vi "Key Join.vi"(11 "Key Elements":string[](array[string])) -> (3 "Key":string)   [LabVIEW 2017]
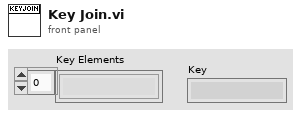
[diagram p1: front panel]
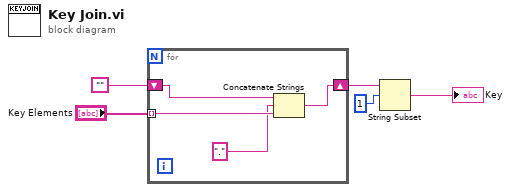
[diagram p0: block diagram]
diagram:
  n1 = for {
    tunnel: "Key Elements" -> [w8] mode=indexing
    shift-right: [w6] -> w3
    shift-left: "" -> [w9]
    n2 = Concatenate Strings(w9, ".", w8) -> (w6:string)
  }
  n3 = String Subset(string=w3, offset (0)=1) -> (substring=→"Key":string)  [unwired: 1 in]
